vi "myFFT_ResultRead.vi"(1 "MultiBuffers 2":T2(array[cluster]), 2 "MultiBuffers 1":T2(array[cluster]), 5 "示波器量程":u16, 6 "可用示波器数":u16, 10 "Max Adc value 2":i16, 11 "Max Adc value":i16) -> (9 "输出簇":T1)   [LabVIEW 2024]
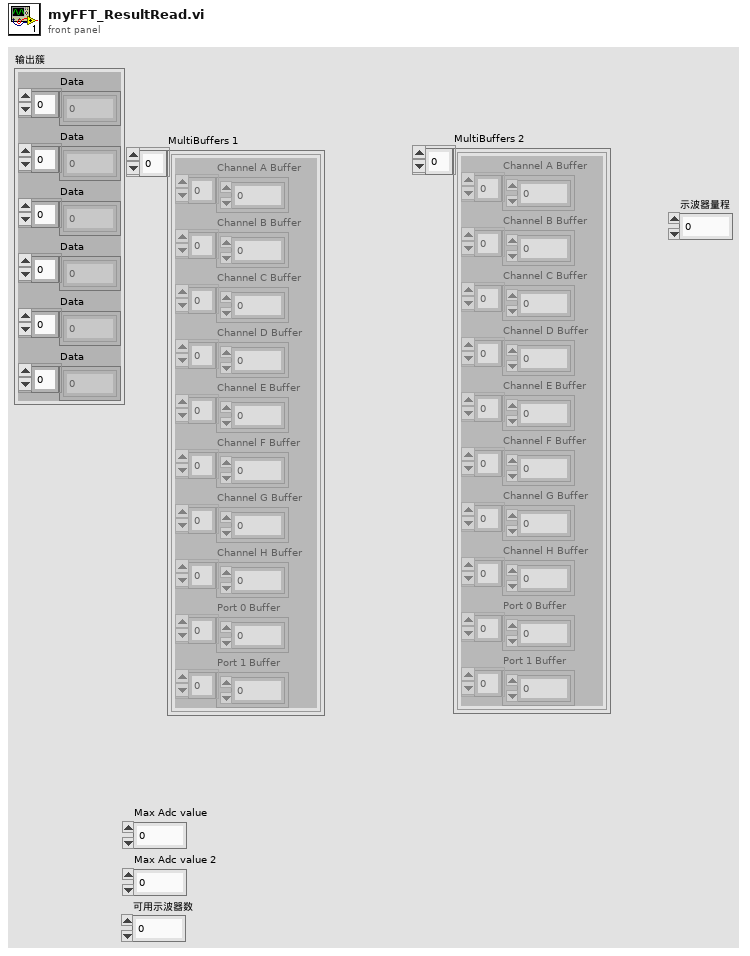
[diagram p1: front panel]
types:
  T1 = cluster{"Data":dbl[], "Data":dbl[], "Data":dbl[], "Data":dbl[], "Data":dbl[], "Data":dbl[]}
  T2 = cluster{"Channel A Buffer":i16[], "Channel B Buffer":i16[], "Channel C Buffer":i16[], "Channel D Buffer":i16[], "Channel E Buffer":i16[], "Channel F Buffer":i16[], "Channel G Buffer":i16[], "Channel H Buffer":i16[], "Port 0 Buffer":i16[], "Port 1 Buffer":i16[]}[]
  T3 = cluster{"Channel A Buffer":i16[], "Channel B Buffer":i16[], "Channel C Buffer":i16[], "Channel D Buffer":i16[], "Channel E Buffer":i16[], "Channel F Buffer":i16[], "Channel G Buffer":i16[], "Channel H Buffer":i16[], "Port 0 Buffer":i16[], "Port 1 Buffer":i16[]}
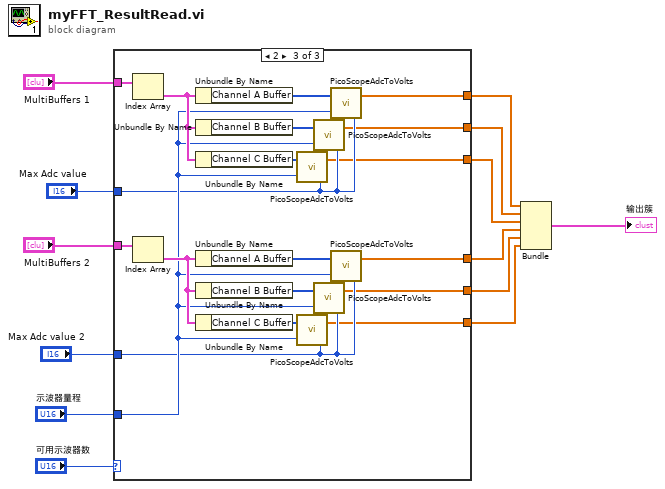
[diagram p0: block diagram]
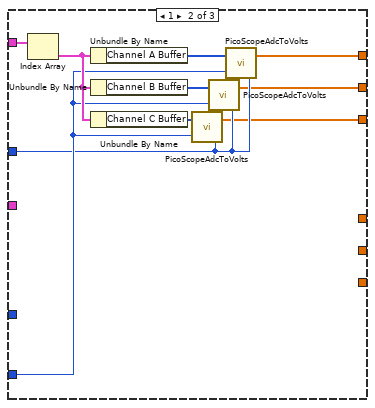
[diagram p3: hidden frame]
diagram:
  n1 = case shown="2" "可用示波器数" {
    tunnel: "MultiBuffers 2" -> [_ _ w34]
    tunnel: "示波器量程" -> [_ w19 w33]
    tunnel: "Max Adc value 2" -> [_ _ w32]
    tunnel: "Max Adc value" -> [_ w18 w31]
    tunnel: "MultiBuffers 1" -> [_ w17 w30]
    tunnel: [_ w16 w29] -> w7
    tunnel: [_ _ w28] -> w2
    tunnel: [_ w15 w27] -> w3
    tunnel: [_ w14 w26] -> w4
    tunnel: [_ _ w25] -> w5
    tunnel: [_ _ w24] -> w6
    frame 0, Default {
    }
    frame 1 {
      n2 = Index Array(array=w17) -> (element=w23:T3)  [unwired: 1 in]
      n3 = Unbundle By Name(w23) -> ("Channel A Buffer"=w21:i16[])
      n4 = Unbundle By Name(w23) -> ("Channel B Buffer"=w22:i16[])
      n5 = Unbundle By Name(w23) -> ("Channel C Buffer"=w20:i16[])
      n6 = call "PicoScopeAdcToVolts.vi"("Max_adc"=w18, "Range Index"=w19, "Data"=w20) -> ("Data"=w14:dbl[])
      n7 = call "PicoScopeAdcToVolts.vi"("Max_adc"=w18, "Range Index"=w19, "Data"=w22) -> ("Data"=w15:dbl[])
      n8 = call "PicoScopeAdcToVolts.vi"("Max_adc"=w18, "Range Index"=w19, "Data"=w21) -> ("Data"=w16:dbl[])
    }
    frame 2 {
      n9 = Index Array(array=w30) -> (element=w42:T3)  [unwired: 1 in]
      n10 = Index Array(array=w34) -> (element=w35:T3)  [unwired: 1 in]
      n11 = Unbundle By Name(w42) -> ("Channel A Buffer"=w40:i16[])
      n12 = Unbundle By Name(w42) -> ("Channel B Buffer"=w41:i16[])
      n13 = Unbundle By Name(w42) -> ("Channel C Buffer"=w39:i16[])
      n14 = Unbundle By Name(w35) -> ("Channel A Buffer"=w37:i16[])
      n15 = Unbundle By Name(w35) -> ("Channel B Buffer"=w36:i16[])
      n16 = Unbundle By Name(w35) -> ("Channel C Buffer"=w38:i16[])
      n17 = call "PicoScopeAdcToVolts.vi"("Max_adc"=w31, "Range Index"=w33, "Data"=w39) -> ("Data"=w26:dbl[])
      n18 = call "PicoScopeAdcToVolts.vi"("Max_adc"=w32, "Range Index"=w33, "Data"=w38) -> ("Data"=w24:dbl[])
      n19 = call "PicoScopeAdcToVolts.vi"("Max_adc"=w31, "Range Index"=w33, "Data"=w41) -> ("Data"=w27:dbl[])
      n20 = call "PicoScopeAdcToVolts.vi"("Max_adc"=w32, "Range Index"=w33, "Data"=w36) -> ("Data"=w25:dbl[])
      n21 = call "PicoScopeAdcToVolts.vi"("Max_adc"=w31, "Range Index"=w33, "Data"=w40) -> ("Data"=w29:dbl[])
      n22 = call "PicoScopeAdcToVolts.vi"("Max_adc"=w32, "Range Index"=w33, "Data"=w37) -> ("Data"=w28:dbl[])
    }
  }
  n23 = Bundle("Data"=w7, "Data"=w3, "Data"=w4, "Data"=w2, "Data"=w5, "Data"=w6) -> (→"输出簇":T1)  [unwired: 1 in]
